vi "sort 2d array.vi"(11 "input":dbl[][](array[numeric])) -> (3 "output":dbl[][](array[numeric]))   [LabVIEW 2014]
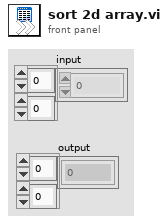
[diagram p1: front panel]
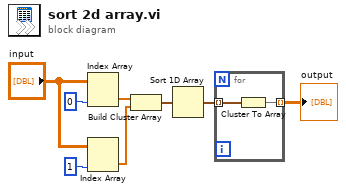
[diagram p0: block diagram]
diagram:
  n1 = Index Array(array="input", index (col)=0 ("disabled index (col)")) -> (element=w4:dbl[])  [unwired: 1 in]
  n2 = Index Array(array="input", index (col)=1 ("disabled index (col)")) -> (element=w5:dbl[])  [unwired: 1 in]
  n3 = Build Cluster Array(w4, w5) -> (w6:cluster{"Numeric":dbl, "Numeric":dbl}[])
  n4 = Sort 1D Array(array=w6) -> (sorted array=w7:cluster{"Numeric":dbl, "Numeric":dbl}[])
  n5 = for {
    tunnel: w7 -> [w10] mode=indexing
    tunnel: [w9] -> w8 mode=indexing
    n6 = Cluster To Array(cluster=w10) -> (array=w9:dbl[])
  }
  "output" <- w8
